vi "Quiz4_TP059851_Sim Yoke Shin_Client.vi"() -> ()   [LabVIEW 2020]
panel:
  in  "Tab Control":enum32{"Page 1", "Page 2"}(tab)
  out "S":bool
  in  "W":bool
  in  "P":bool
  in  "T":bool
  # "Client"
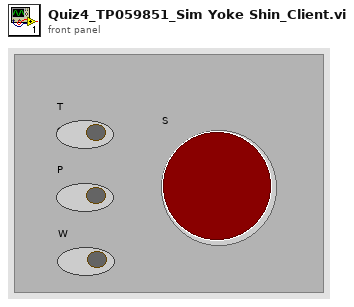
[diagram p1: front panel]
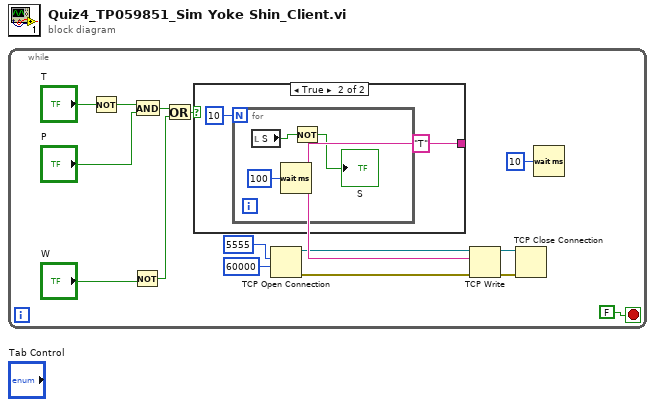
[diagram p0: block diagram]
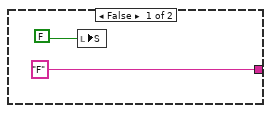
[diagram p2: hidden frame]
diagram:
  n1 = while {
    stop <- FALSE stop-if-true
    n2 = Not(x="T") -> (.not. x?=w12:bool)
    n3 = Not(x="W") -> (.not. x?=w15:bool)
    n4 = And(x=w12, y="P") -> (x .and. y?=w10:bool)
    n5 = Or(x=w10, y=w15) -> (x .or. y?=w5:bool)
    n6 = case shown="True" w5 {
      tunnel: ["F" "T"] -> w4
      frame False {
        n7 = local write "S"(FALSE ("S")) -> ()
      }
      frame True {
        n8 = for {
          N: 10 -> [_]
          n9 = local read "S"() -> (w23:bool)
          n10 = Wait (ms)(milliseconds to wait=u32 100) -> ()  [unwired: 1 out]
          n11 = Not(x=w23) -> (.not. x?=→"S":bool)
        }
      }
    }
    n12 = TCP Open Connection(remote port or service name=u16 5555, timeout ms (60000)=60000) -> (connection ID=w3:refnum<k5>, error out=w2:errorcluster)  [unwired: 3 in]
    n13 = TCP Write(connection ID=w3, data in=w4, error in (no error)=w2) -> (connection ID out=w9:refnum<k5>, error out=w8:errorcluster)  [unwired: 1 in, 1 out]
    n14 = TCP Close Connection(connection ID=w9, error in (no error)=w8) -> ()  [unwired: 1 in, 2 out]
    n15 = Wait (ms)(milliseconds to wait=u32 10) -> ()  [unwired: 1 out]
  }
